vi "PDW gen.vi"() -> ()   [LabVIEW 2021]
uses:
  emitter params.ctl
  <vilib>/numeric/Random Number (Range) U64.vi
  <vilib>/numeric/Random Number (Range) DBL.vi
  <vilib>/numeric/sub_Random U32.vi
panel:
  out "may saturate":bool
  out "sorted array":T1(array[cluster])
  in  "start time":dbl format="%#_13g"
  out "num of pulses":i32=44546
  in  "num of frequncys upper bound":u64=15
  in  "num of frequncys type lower":u64=1
  in  "f mode depth  lower bound":dbl=2000000.0
  in  "f mode depth upper bound":dbl=10000000.0
  in  "mode file upper bound":u64=3
  in  "mode file lower":u64
  in  "mode type lower":u64
  in  "mode type upper bound":u64=3
  in  "Fs":i32=200000000 format="%.0p"
  in  "tdms output file path":path=path "C:/Users/NI/Documents/chaim/chaim_rx/chaim_data/pulses.tdms"
  in  "secnario length (sec)":dbl=50.0
  out "emmiters array":T2[](array[typedef])=[{"f set"=[10000000.0], "hop rate (Hz)"=1.0, "d.c."=0.999, "amp (dB)"=-5.0, "mod type"=4, "mod file 2"=0, "mod depth"=1000000.0}, {"f set"=[40000000.0], "hop rate (Hz)"=1.0, "d.c."=0.999, "amp (dB)"=-5.0, "mod type"=5, "mod file 2"=0, "mod depth"=100000.0}, {"f set"=[-15312834.181529276, -17093032.382574577, -17146959.37176916, -16650115.792208051, -15721755.611738132, -17159986.21721435, -16204297.424796015, -16724918.0939007, -17157934.36678599, -16888086.283555575], "hop rate (Hz)"=241.66649372638219, "d.c."=0.8105375049871737, "amp (dB)"=-29.29304171093305, "mod type"=0, "mod file 2"=1, "mod depth"=9937990.796627652}, {"f set"=[-11491406.539901216, -9953009.420672901, -10722698.354196433, -10078675.887961177, -12862181.660160841, -10128405.860170962, -10719720.984941227, -11073798.957973663, -11505970.074857479, -12496118.546890486], "hop rate (Hz)"=245.14157663855235, "d.c."=0.8708349033890386, "amp (dB)"=-29.048710424249357, "mod type"=3, "mod file 2"=3, "mod depth"=8098552.870862729}, {"f set"=[-6775828.497782527, -3303786.73430779, -4884777.271048309, -6298131.646679702, 323498.28385398537, 1478431.3018701999, 1112783.099566943, -4734067.158852352, -5402897.305479352, 1611615.3212139262, 1725261.2042662138], "hop rate (Hz)"=229.52551792917814, "d.c."=0.7429543671055145, "amp (dB)"=-11.574753843465544, "mod type"=0, "mod file 2"=2, "mod depth"=2537362.6471950673}, {"f set"=[-74109065.64272028, -68519180.44095898, -71794296.98663852, -72976696.59705997, -74040765.7303411, -71428888.24437326, -72291156.6916291, -72220283.69245422], "hop rate (Hz)"=172.49647059892766, "d.c."=0.74263129942552, "amp (dB)"=-27.149219397826645, "mod type"=3, "mod file 2"=3, "mod depth"=3914870.3065856127}] {"hop rate (Hz)" format="%#_3p"}
  in  "span  lower bound":dbl=2000000.0
  in  "span upper bound":dbl=10000000.0
  in  "f band  lower bound":dbl=-80000000.0
  in  "f band upper bound":dbl
  in  "amp  lower bound":dbl=-15.0
  in  "amp upper bound":dbl=-5.0
  in  "D C upper bound":dbl=0.98
  in  "D C lower bound":dbl=0.7000000000000001
  in  "HR lower bound":dbl=150.0
  in  "HR upper bound":dbl=300.0
  in  "user bulid emmiters":T2[](array[typedef])=[{"f set"=[10000000.0], "hop rate (Hz)"=1.0, "d.c."=0.999, "amp (dB)"=-5.0, "mod type"=4, "mod file 2"=0, "mod depth"=1000000.0}, {"f set"=[40000000.0], "hop rate (Hz)"=1.0, "d.c."=0.999, "amp (dB)"=-5.0, "mod type"=5, "mod file 2"=0, "mod depth"=100000.0}] {"mod depth" format="%#_6p"}
  in  "auto gen num of nets":i32=4
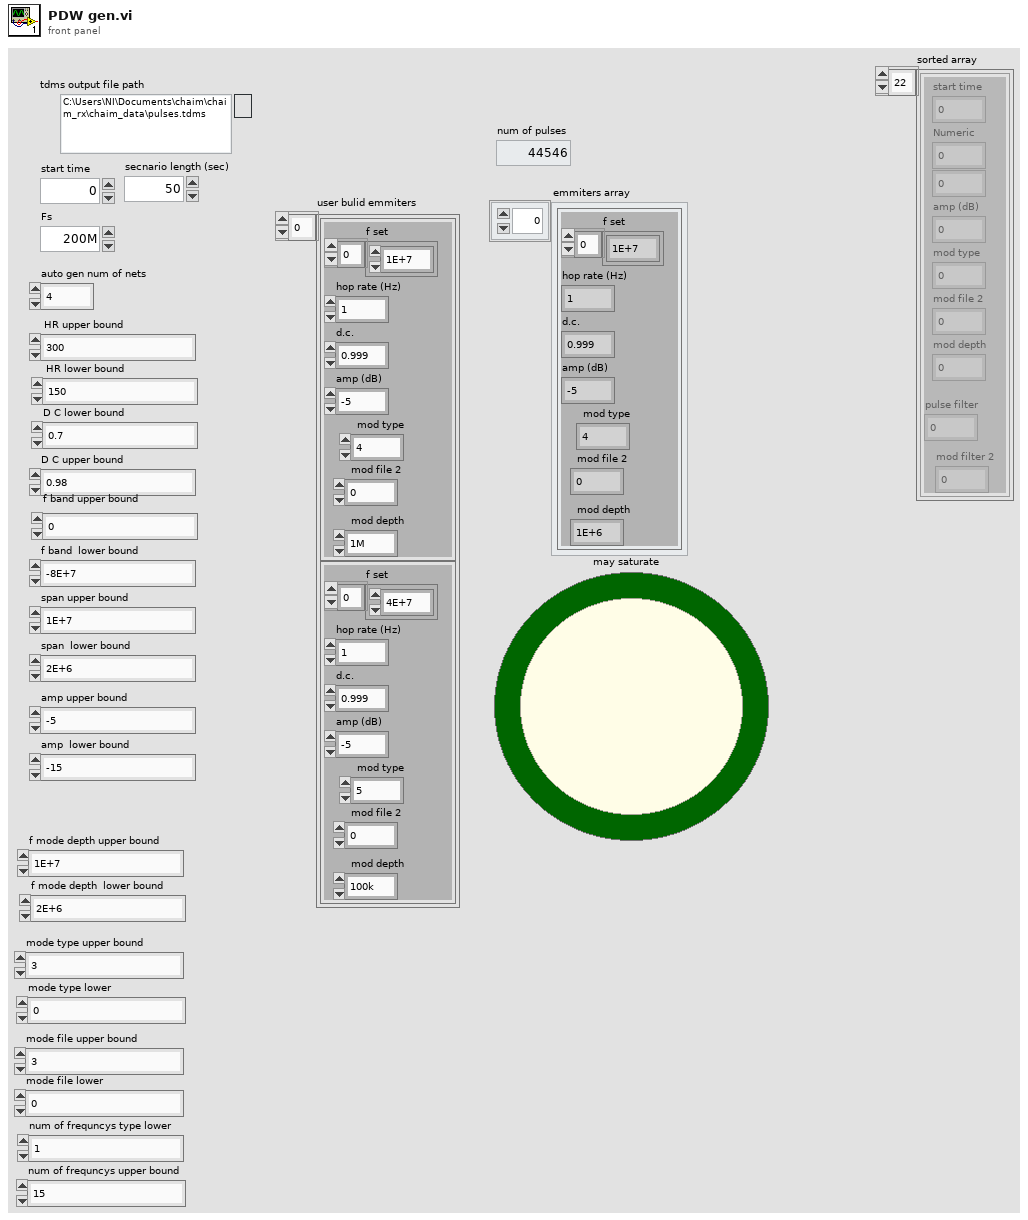
[diagram p1: front panel]
types:
  T1 = cluster{"start time":dbl, "Numeric":dbl, dbl, "amp (dB)":dbl, "mod type":u8, "mod file 2":u8, "mod depth":dbl, "pulse filter":u16, "mod filter 2":u16}[]
  T2 = typedef "emitter params.ctl" = cluster{"f set":dbl[], "hop rate (Hz)":dbl, "d.c.":dbl, "amp (dB)":dbl, "mod type":u8, "mod file 2":u8, "mod depth":dbl}
  T3 = enum16{"open", "open or create", "create or replace", "create", "open (read-only)"}
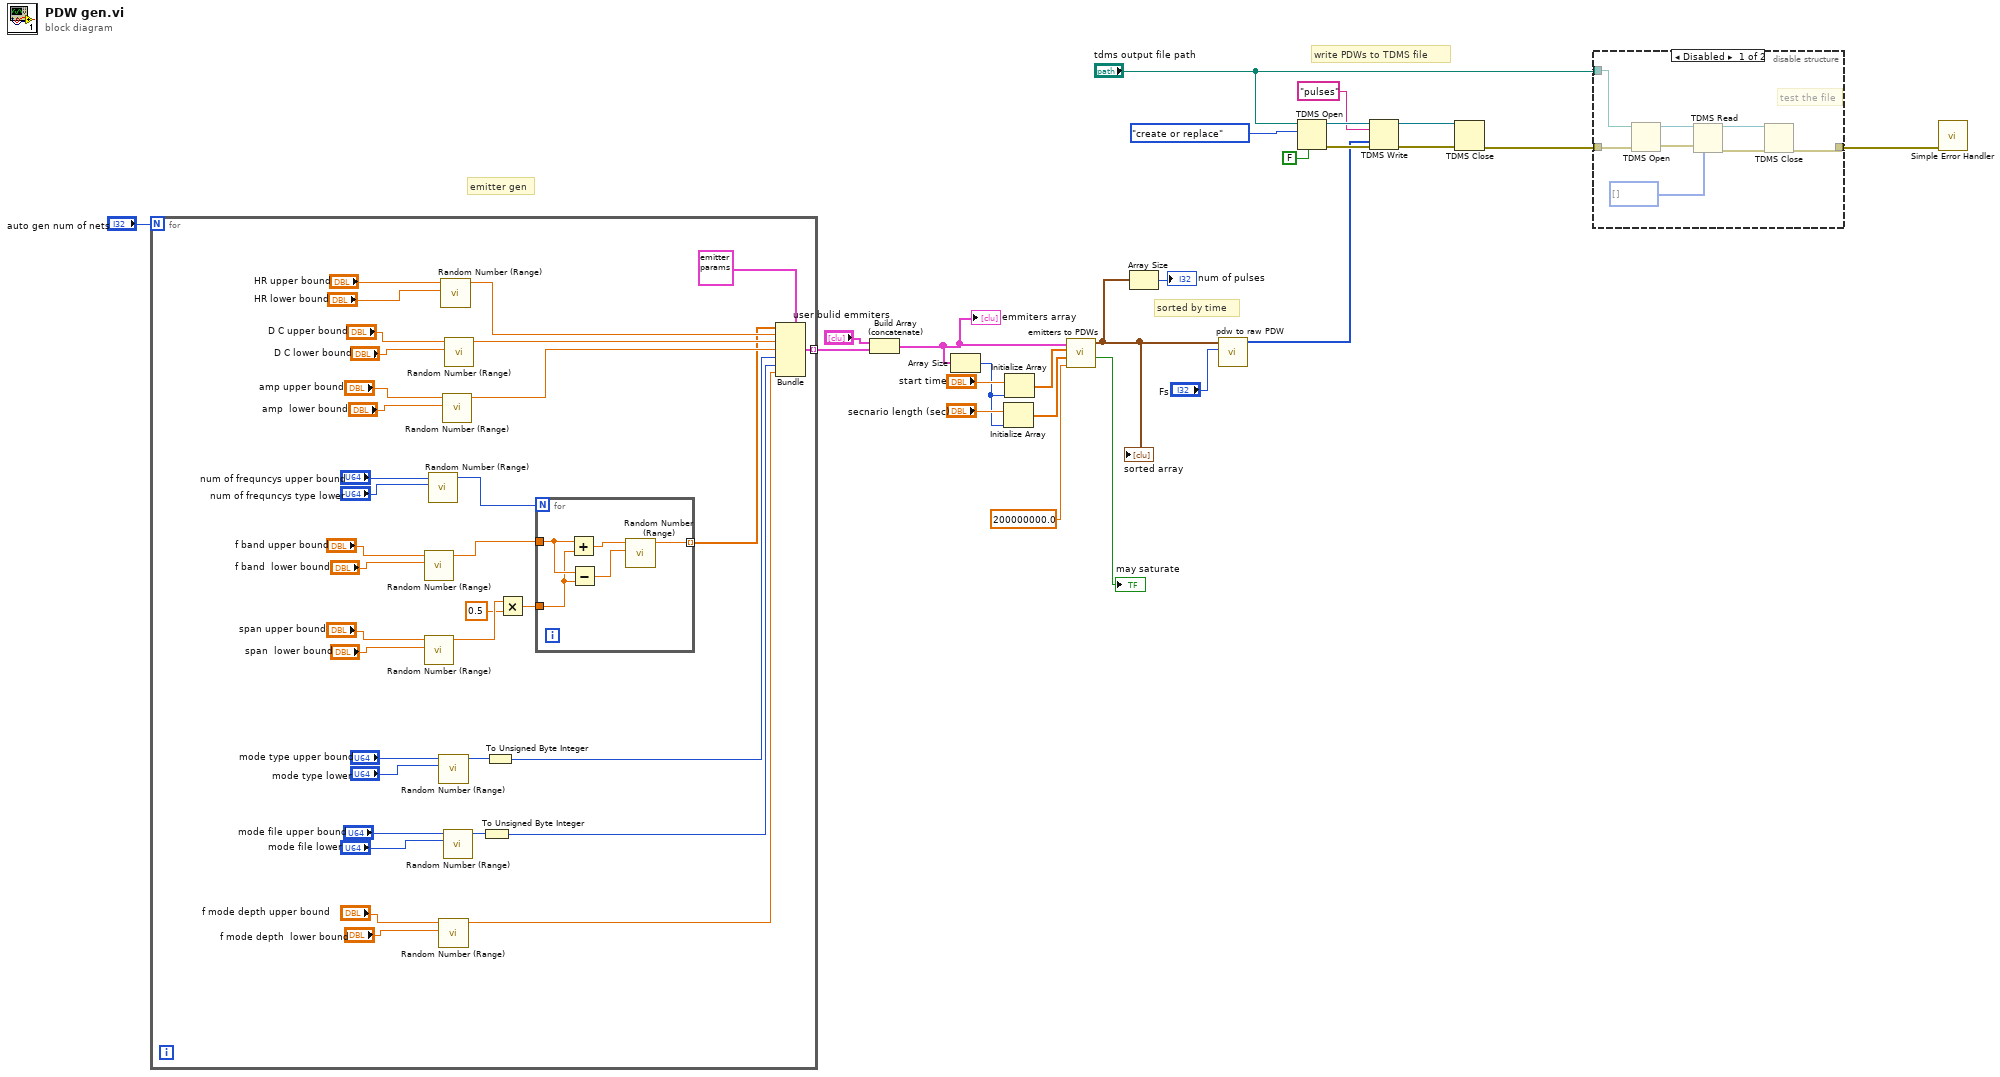
[diagram p0: block diagram]
diagram:
  # "write PDWs to TDMS file"
  # "sorted by time"
  # "emitter gen"
  n1 = for {
    N: "auto gen num of nets" -> [_]
    tunnel: [w40] -> w23 mode=indexing
    n2 = call-poly <vilib>:"Random Number (Range).vi"("lower bound (0)"="f band  lower bound", "upper bound (100)"="f band upper bound") -> ("number"=w43:dbl)  [unwired: 9 in]
    n3 = call-poly <vilib>:"Random Number (Range).vi"("lower bound (0)"="span  lower bound", "upper bound (100)"="span upper bound") -> ("number"=w45:dbl)  [unwired: 9 in]
    n4 = call-poly <vilib>:"Random Number (Range).vi"("lower bound (0)"="num of frequncys type lower", "upper bound (100)"="num of frequncys upper bound") -> ("number"=w26:u64)  [unwired: 9 in]
    n5 = call-poly <vilib>:"Random Number (Range).vi"("lower bound (0)"="mode type lower", "upper bound (100)"="mode type upper bound") -> ("number"=w35:u64)  [unwired: 9 in]
    n6 = call-poly <vilib>:"Random Number (Range).vi"("lower bound (0)"="f mode depth  lower bound", "upper bound (100)"="f mode depth upper bound") -> ("number"=w29:dbl)  [unwired: 9 in]
    n7 = call-poly <vilib>:"Random Number (Range).vi"("lower bound (0)"="HR lower bound", "upper bound (100)"="HR upper bound") -> ("number"=w56:dbl)  [unwired: 9 in]
    n8 = call-poly <vilib>:"Random Number (Range).vi"("lower bound (0)"="amp  lower bound", "upper bound (100)"="amp upper bound") -> ("number"=w51:dbl)  [unwired: 9 in]
    n9 = call-poly <vilib>:"Random Number (Range).vi"("lower bound (0)"="mode file lower", "upper bound (100)"="mode file upper bound") -> ("number"=w34:u64)  [unwired: 9 in]
    n10 = call-poly <vilib>:"Random Number (Range).vi"("lower bound (0)"="D C lower bound", "upper bound (100)"="D C upper bound") -> ("number"=w55:dbl)  [unwired: 9 in]
    n11 = To Unsigned Byte Integer(number=w34) -> (unsigned 8bit integer=w32:u8)
    n12 = To Unsigned Byte Integer(number=w35) -> (unsigned 8bit integer=w33:u8)
    n13 = Multiply(x=w45, y=0.5) -> (x*y=w42:dbl)
    n14 = for {
      N: w26 -> [_]
      tunnel: w43 -> [w64]
      tunnel: w42 -> [w63]
      tunnel: [w60] -> w41 mode=indexing
      n15 = Add(x=w64, y=w63) -> (x+y=w61:dbl)
      n16 = Subtract(x=w64, y=w63) -> (x-y=w62:dbl)
      n17 = call-poly <vilib>:"Random Number (Range).vi"("lower bound (0)"=w62, "upper bound (100)"=w61) -> ("number"=w60:dbl)  [unwired: 9 in]
    }
    n18 = Bundle(cluster=T2 {"f set"=[1000000.0], "hop rate (Hz)"=300000.0, "d.c."=0.0, "amp (dB)"=-20.0, "mod type"=0, "mod file 2"=0, "mod depth"=0.0} ("Cluster"), "f set"=w41, "hop rate (Hz)"=w56, "d.c."=w55, "amp (dB)"=w51, "mod type"=w33, "mod file 2"=w32, "mod depth"=w29) -> (w40:T2)
  }
  n19 = Build Array (concatenate)("user bulid emmiters", w23) -> (w9:T2[])
  "emmiters array" <- w9
  n20 = Array Size(array=w9) -> (size(s)=w6:i32)
  n21 = Initialize Array("secnario length (sec)", w6) -> (w4:dbl[])
  n22 = Initialize Array("start time", w6) -> (w5:dbl[])
  n23 = call "emitters to PDWs.vi"("fs [Hz]"=200000000.0, "end time"=w4, "start time"=w5, "emmiter"=w9) -> ("my saturate"=→"may saturate":bool, "sorted array"=w11:T1)  [unwired: 6 in]
  "sorted array" <- w11
  n24 = Array Size(array=w11) -> (size(s)=→"num of pulses":i32)
  n25 = call "pdw to raw PDW.vi"("Fs"="Fs", "PDW"=w11) -> ("Array"=w13:u64[])  [unwired: 9 in]
  n26 = TDMS Open(6:FALSE ("enable asynchronous? (T)"), 10:T3."create or replace" ("operation (0:open)"), 11:"tdms output file path") -> (0:w20:errorcluster, 3:w17:refnum<k34>)  [unwired: 4 in]
  n27 = TDMS Write(0:w17, 5:"pulses" ("group name in (Untitled)"), 9:w13, 11:w20) -> (4:w22:refnum<k34>, 15:w21:errorcluster)  [unwired: 2 in, 2 out]
  n28 = TDMS Close(8:w21, 11:w22) -> (0:w14:errorcluster)  [unwired: 1 out]
  n29 = disable-structure "Diagram Disable Structure" shown="Disabled" {
    disable-tunnel: "tdms output file path" -> [w69 _]
    disable-tunnel: w14 -> [w66 w73]
    disable-tunnel: [w65 w73] -> w3
    frame Disabled {
      # "test the file"
      n30 = TDMS Open(8:w66, 11:w69) -> (0:w71:errorcluster, 3:w68:refnum<k34>)  [unwired: 5 in]
      n31 = TDMS Read(0:w68, 11:w71, 12:u64[] [] ("Data")) -> (4:w67:refnum<k34>, 15:w70:errorcluster)  [unwired: 5 in, 4 out]
      n32 = TDMS Close(8:w70, 11:w67) -> (0:w65:errorcluster)  [unwired: 1 out]
    }
    frame Enabled {
    }
  }
  n33 = call <vilib>:"Simple Error Handler.vi"("error in (no error)"=w3) -> ()  [unwired: 4 in, 5 out]
